vi "Image_Folder_Path_Checker.vi"(11 "Path":path) -> (3 "appended path":path)   [LabVIEW 2024]
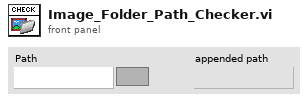
[diagram p1: front panel]
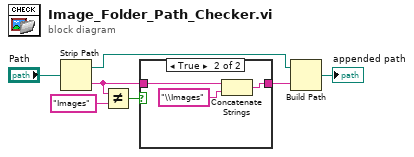
[diagram p0: block diagram]
diagram:
  n1 = Strip Path(path="Path") -> (stripped path=w4:path, name=w3:string)
  n2 = Not Equal?(x=w3, y="Images") -> (x != y?=w2:bool)
  n3 = case shown="True" w2 {
    tunnel: w3 -> [w8 w11]
    tunnel: [w8 w9] -> w5
    frame False {
    }
    frame True {
      n4 = Concatenate Strings(w11, "\\Images" ("string")) -> (w9:string)
    }
  }
  n5 = Build Path(base path=w4, name or relative path=w5) -> (appended path=→"appended path":path)
